vi "example_asynch_wait_1.vi"() -> ()   [LabVIEW 2015]
uses:
  polys/poly_now_ms_timer.vi
  polys/poly_asynch_wait_wait.vi
  cores/core_timing_tools_eco.vi
  polys/poly_timing_tools_eco_plus.vi
  ref_tools/name_of_caller.vi
  cast_boolean_notifier.vi
  polys/poly_cast_boolean_notifier_n2q.vi
  polys/poly_cast_boolean_notifier_q2n.vi
  polys/poly_asynch_wait_start.vi
  polys/poly_asynch_wait_notify.vi
  polys/poly_asynch_wait_stop.vi
  loop_timeout.vi
  polys/poly_loop_timeout_bool.vi
  error_tools/merge_errors.vi
  error_tools/polys/poly_merge_errors_down.vi
  error_tools/toolbox_error_handler.vi
  <vilib>/Utility/error.llb/Simple Error Handler.vi
panel:
  out "4 wait time":u32
  out "3 wait time":u32
  out "2 wait time":u32
  out "1 wait time":u32
  in  "stop":bool
  out "4 name":string
  out "3 name":string
  out "2 name":string
  out "1 name":string
  in  "4 stop":bool
  in  "3 stop":bool
  in  "2 stop":bool
  in  "4 notify":bool
  in  "3 notify":bool
  in  "2 notify":bool
  in  "4 timeout":i32=-1 format="%.0f ms"
  in  "3 timeout":i32=3000 format="%.0f ms"
  in  "2 timeout":i32=2000 format="%.0f ms"
  in  "1 timeout":i32=1000 format="%.0f ms"
  in  "1 stop":bool
  in  "1 notify":bool
  out "4 error":bool
  out "3 error":bool
  out "2 error":bool
  out "1 error":bool
  out "4 timeout":bool
  out "3 timeout":bool
  out "2 timeout":bool
  out "1 tiemout":bool
  out "4 done":bool
  out "3 done":bool
  out "2 done":bool
  out "1 done":bool
  # "notifier names"
  # "timeout [ms]"
  # "done"
  # "timed out"
  # "error"
  # "send notif."
  # "stop"
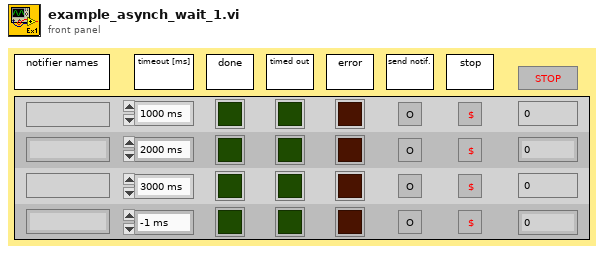
[diagram p1: front panel]
types:
  T1 = typedef "boolean_notifier.ctl" = refnum<k1>
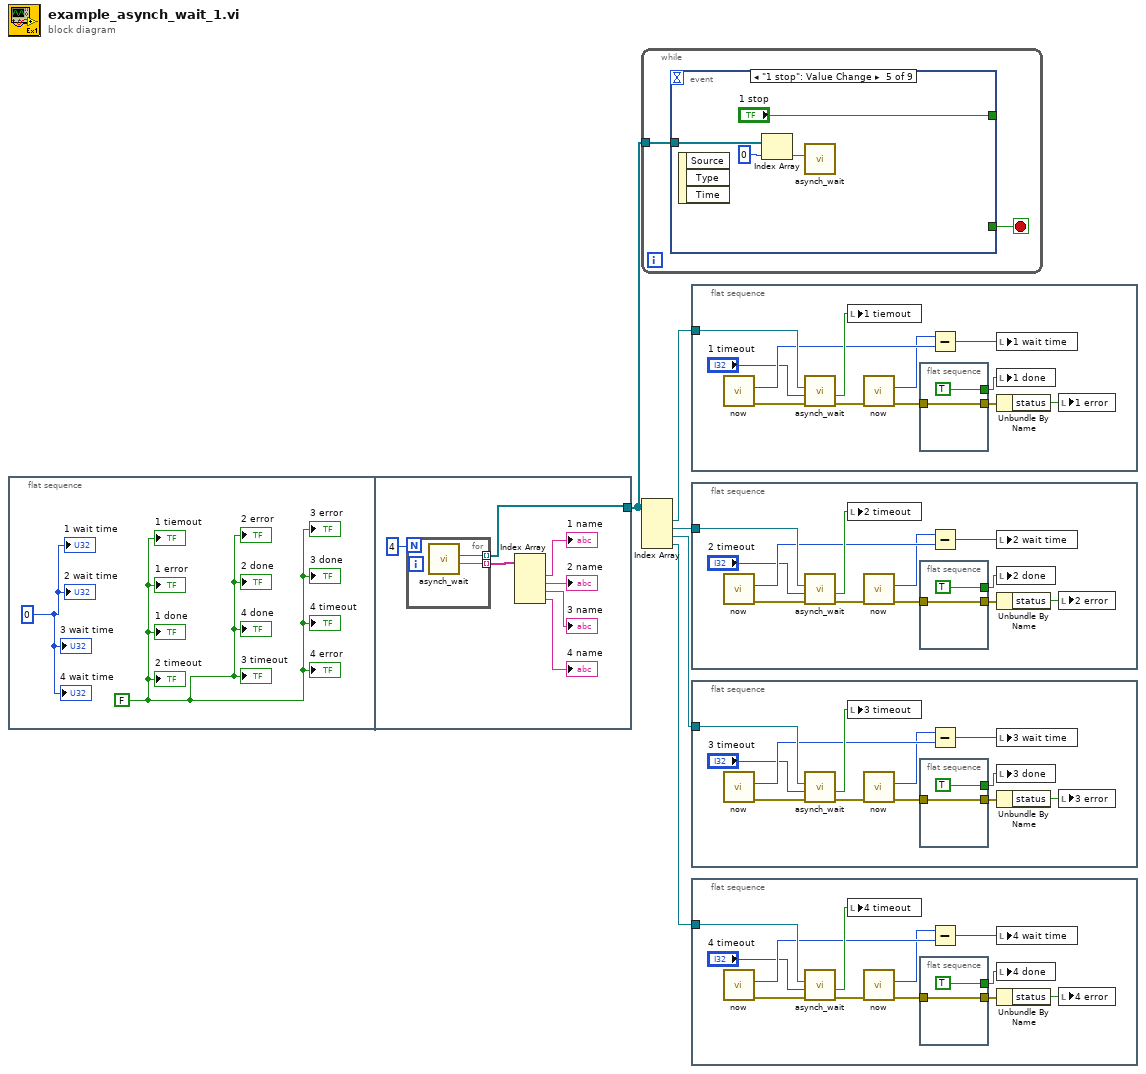
[diagram p0: block diagram]
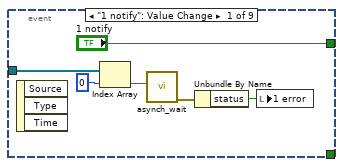
[diagram p2: hidden frame]
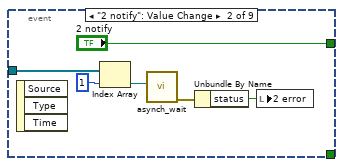
[diagram p3: hidden frame]
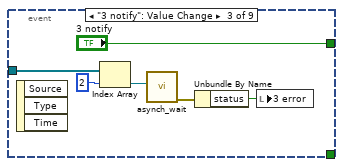
[diagram p4: hidden frame]
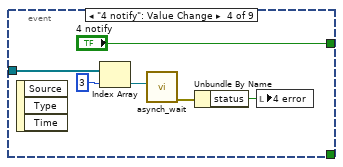
[diagram p5: hidden frame]
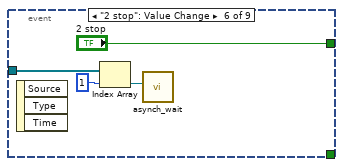
[diagram p6: hidden frame]
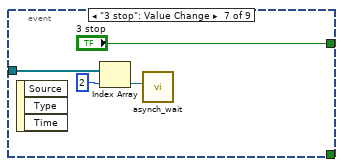
[diagram p7: hidden frame]
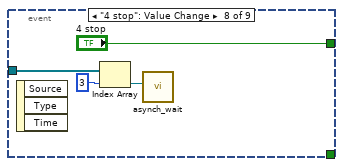
[diagram p8: hidden frame]
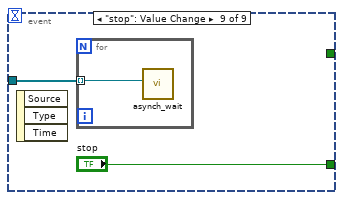
[diagram p9: hidden frame]
diagram:
  n1 = flat-sequence {
    tunnel: [w9] -> w1
    frame #0 {
      w7 = FALSE
      w6 = u32 0
      "1 done" <- w7
      "2 done" <- w7
      "3 done" <- w7
      "4 done" <- w7
      "1 tiemout" <- w7
      "2 timeout" <- w7
      "3 timeout" <- w7
      "4 timeout" <- w7
      "1 error" <- w7
      "2 error" <- w7
      "3 error" <- w7
      "4 error" <- w7
      "1 wait time" <- w6
      "2 wait time" <- w6
      "3 wait time" <- w6
      "4 wait time" <- w6
    }
    frame #1 {
      n2 = for {
        N: 4 -> [_]
        tunnel: [w15] -> w10 mode=indexing
        tunnel: [w16] -> w9 mode=indexing
        n3 = call-poly "asynch_wait.vi"() -> ("notifier name"=w15:string, "notifier"=w16:T1)  [unwired: 9 in, 1 out]
      }
      n4 = Index Array(array=w10) -> (element #1=→"1 name":string, element #2=→"2 name":string, element #3=→"3 name":string, element #4=→"4 name":string)  [unwired: 4 in]
    }
  }
  n5 = while {
    tunnel: w1 -> [w18]
    stop <- w17 stop-if-true
    n6 = event shown="[4] \"1 stop\": Value Change" {
      selector: _ -> [_ _ _ _ _ _ _ _ _]
      dyn-events: _ -> [_ _ _ _ _ _ _ _ _]
      timeout: _ -> [_ _ _ _ _ _ _ _ _]
      tunnel: w18 -> [w24 w30 w36 w42 w46 w50 w54 w58 w59]
      tunnel: ["1 notify" "2 notify" "3 notify" "4 notify" "1 stop" "2 stop" "3 stop" "4 stop" _] -> _
      tunnel: [_ _ _ _ _ _ _ _ "stop"] -> w17
      event "1 notify": Value Change {
        n7 = event-data() -> ()  [unwired: 1 in, 3 out]
        n8 = Index Array(array=w24, index=0) -> (element=w21:T1)
        n9 = call-poly "asynch_wait.vi"("notifier"=w21) -> ("error out"=w19:errorcluster)  [unwired: 9 in, 1 out]
        n10 = Unbundle By Name(w19) -> ("status"=w20:bool)
        n11 = local write "1 error"(w20) -> ()
      }
      event "2 notify": Value Change {
        n12 = event-data() -> ()  [unwired: 1 in, 3 out]
        n13 = Index Array(array=w30, index=1) -> (element=w27:T1)
        n14 = call-poly "asynch_wait.vi"("notifier"=w27) -> ("error out"=w25:errorcluster)  [unwired: 9 in, 1 out]
        n15 = Unbundle By Name(w25) -> ("status"=w26:bool)
        n16 = local write "2 error"(w26) -> ()
      }
      event "3 notify": Value Change {
        n17 = event-data() -> ()  [unwired: 1 in, 3 out]
        n18 = Index Array(array=w36, index=2) -> (element=w33:T1)
        n19 = call-poly "asynch_wait.vi"("notifier"=w33) -> ("error out"=w31:errorcluster)  [unwired: 9 in, 1 out]
        n20 = Unbundle By Name(w31) -> ("status"=w32:bool)
        n21 = local write "3 error"(w32) -> ()
      }
      event "4 notify": Value Change {
        n22 = event-data() -> ()  [unwired: 1 in, 3 out]
        n23 = Index Array(array=w42, index=3) -> (element=w39:T1)
        n24 = call-poly "asynch_wait.vi"("notifier"=w39) -> ("error out"=w37:errorcluster)  [unwired: 9 in, 1 out]
        n25 = Unbundle By Name(w37) -> ("status"=w38:bool)
        n26 = local write "4 error"(w38) -> ()
      }
      event "1 stop": Value Change {
        n27 = event-data() -> ()  [unwired: 1 in, 3 out]
        n28 = Index Array(array=w46, index=0) -> (element=w44:T1)
        n29 = call-poly "asynch_wait.vi"("notifier"=w44) -> ()  [unwired: 10 in, 1 out]
      }
      event "2 stop": Value Change {
        n30 = event-data() -> ()  [unwired: 1 in, 3 out]
        n31 = Index Array(array=w50, index=1) -> (element=w48:T1)
        n32 = call-poly "asynch_wait.vi"("notifier"=w48) -> ()  [unwired: 10 in, 1 out]
      }
      event "3 stop": Value Change {
        n33 = event-data() -> ()  [unwired: 1 in, 3 out]
        n34 = Index Array(array=w54, index=2) -> (element=w52:T1)
        n35 = call-poly "asynch_wait.vi"("notifier"=w52) -> ()  [unwired: 10 in, 1 out]
      }
      event "4 stop": Value Change {
        n36 = event-data() -> ()  [unwired: 1 in, 3 out]
        n37 = Index Array(array=w58, index=3) -> (element=w56:T1)
        n38 = call-poly "asynch_wait.vi"("notifier"=w56) -> ()  [unwired: 10 in, 1 out]
      }
      event "stop": Value Change {
        n39 = event-data() -> ()  [unwired: 1 in, 3 out]
        n40 = for {
          tunnel: w59 -> [w61] mode=indexing
          n41 = call-poly "asynch_wait.vi"("notifier"=w61) -> ()  [unwired: 10 in, 1 out]
        }
      }
    }
  }
  n42 = Index Array(array=w1) -> (element #1=w5:T1, element #2=w4:T1, element #3=w3:T1, element #4=w2:T1)  [unwired: 4 in]
  n43 = flat-sequence {
    tunnel: w5 -> [w73]
    frame #0 {
      n44 = call-poly "now.vi"() -> ("Error out"=w66:errorcluster, "millisecond timer value"=w67:i32)  [unwired: 10 in]
      n45 = call-poly "asynch_wait.vi"("error in"=w66, "timeout"="1 timeout", "notifier"=w73) -> ("error out"=w65:errorcluster, "timed out?"=w72:bool)  [unwired: 6 in, 1 out]
      n46 = local write "1 tiemout"(w72) -> ()
      n47 = call-poly "now.vi"("Error in"=w65) -> ("Error out"=w63:errorcluster, "millisecond timer value"=w64:i32)  [unwired: 9 in]
      n48 = flat-sequence {
        tunnel: [TRUE] -> w69
        tunnel: [w74] -> w70
        tunnel: w63 -> [w74]
        frame #0 {
        }
      }
      n49 = Subtract(x=w64, y=w67) -> (x-y=w68:i32)
      n50 = local write "1 wait time"(w68) -> ()
      n51 = local write "1 done"(w69) -> ()
      n52 = Unbundle By Name(w70) -> ("status"=w71:bool)
      n53 = local write "1 error"(w71) -> ()
    }
  }
  n54 = flat-sequence {
    tunnel: w4 -> [w87]
    frame #0 {
      n55 = call-poly "now.vi"() -> ("Error out"=w80:errorcluster, "millisecond timer value"=w81:i32)  [unwired: 10 in]
      n56 = call-poly "asynch_wait.vi"("error in"=w80, "timeout"="2 timeout", "notifier"=w87) -> ("error out"=w79:errorcluster, "timed out?"=w86:bool)  [unwired: 6 in, 1 out]
      n57 = local write "2 timeout"(w86) -> ()
      n58 = call-poly "now.vi"("Error in"=w79) -> ("Error out"=w77:errorcluster, "millisecond timer value"=w78:i32)  [unwired: 9 in]
      n59 = flat-sequence {
        tunnel: [TRUE] -> w83
        tunnel: [w88] -> w84
        tunnel: w77 -> [w88]
        frame #0 {
        }
      }
      n60 = Subtract(x=w78, y=w81) -> (x-y=w82:i32)
      n61 = local write "2 wait time"(w82) -> ()
      n62 = local write "2 done"(w83) -> ()
      n63 = Unbundle By Name(w84) -> ("status"=w85:bool)
      n64 = local write "2 error"(w85) -> ()
    }
  }
  n65 = flat-sequence {
    tunnel: w3 -> [w101]
    frame #0 {
      n66 = call-poly "now.vi"() -> ("Error out"=w95:errorcluster, "millisecond timer value"=w94:i32)  [unwired: 10 in]
      n67 = call-poly "asynch_wait.vi"("error in"=w95, "timeout"="3 timeout", "notifier"=w101) -> ("error out"=w93:errorcluster, "timed out?"=w100:bool)  [unwired: 6 in, 1 out]
      n68 = local write "3 timeout"(w100) -> ()
      n69 = call-poly "now.vi"("Error in"=w93) -> ("Error out"=w91:errorcluster, "millisecond timer value"=w92:i32)  [unwired: 9 in]
      n70 = flat-sequence {
        tunnel: [TRUE] -> w97
        tunnel: [w102] -> w98
        tunnel: w91 -> [w102]
        frame #0 {
        }
      }
      n71 = Subtract(x=w92, y=w94) -> (x-y=w96:i32)
      n72 = local write "3 wait time"(w96) -> ()
      n73 = local write "3 done"(w97) -> ()
      n74 = Unbundle By Name(w98) -> ("status"=w99:bool)
      n75 = local write "3 error"(w99) -> ()
    }
  }
  n76 = flat-sequence {
    tunnel: w2 -> [w112]
    frame #0 {
      n77 = call-poly "now.vi"() -> ("Error out"=w109:errorcluster, "millisecond timer value"=w108:i32)  [unwired: 10 in]
      n78 = call-poly "asynch_wait.vi"("error in"=w109, "timeout"="4 timeout", "notifier"=w112) -> ("error out"=w107:errorcluster, "timed out?"=w114:bool)  [unwired: 6 in, 1 out]
      n79 = local write "4 timeout"(w114) -> ()
      n80 = call-poly "now.vi"("Error in"=w107) -> ("Error out"=w106:errorcluster, "millisecond timer value"=w105:i32)  [unwired: 9 in]
      n81 = flat-sequence {
        tunnel: [TRUE] -> w115
        tunnel: [w116] -> w111
        tunnel: w106 -> [w116]
        frame #0 {
        }
      }
      n82 = Subtract(x=w105, y=w108) -> (x-y=w110:i32)
      n83 = local write "4 wait time"(w110) -> ()
      n84 = local write "4 done"(w115) -> ()
      n85 = Unbundle By Name(w111) -> ("status"=w113:bool)
      n86 = local write "4 error"(w113) -> ()
    }
  }
